vi "ConvertImage.vi"(11 "body":string) -> (3 "new picture":picture)   [LabVIEW 2019]
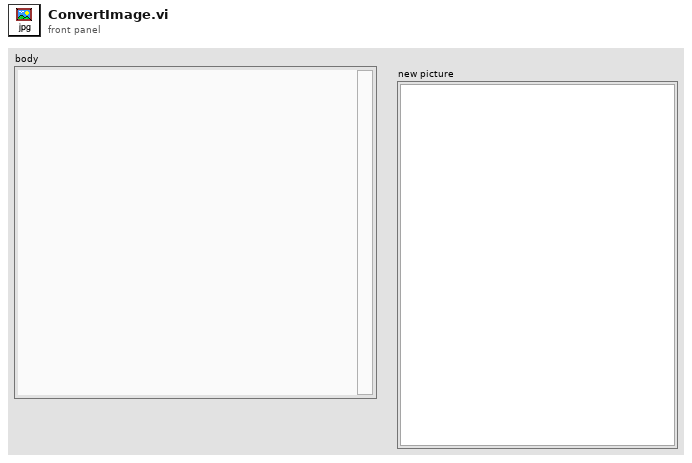
[diagram p1: front panel]
types:
  T1 = typedef "imagedata.ctl" = cluster{"image type":i32, "image depth":i32, "image":u8[], "mask":u8[], "colors":u32[], "Rectangle":cluster{"left":i16, "top":i16, "right":i16, "bottom":i16}}
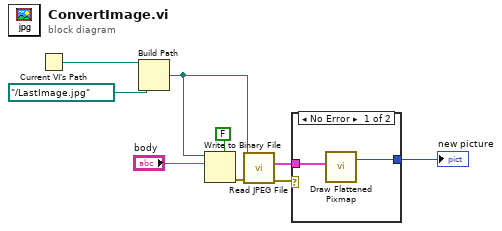
[diagram p0: block diagram]
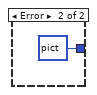
[diagram p2: hidden frame]
diagram:
  n1 = Current VI's Path() -> (path=w3:path)
  n2 = Build Path(base path=w3, name or relative path=path "../LastImage.jpg") -> (appended path=w2:path)
  n3 = Write to Binary File(file (use dialog)=w2, data="body", 5:FALSE ("prepend array or string size? (T)")) -> (error out=w9:errorcluster)  [unwired: 3 in, 2 out]
  n4 = call <vilib>:"Read JPEG File.vi"("error in (no error)"=w9, "path to JPEG file"=w2) -> ("error out"=w4:errorcluster, "image data"=w5:T1)  [unwired: 7 in, 1 out]
  n5 = case shown="No Error" w4 {
    tunnel: [w11 picture data[5B] ("new picture")] -> w7
    tunnel: w5 -> [w10 _]
    frame No Error {
      n6 = call <vilib>:"Draw Flattened Pixmap.vi"("image data"=w10) -> ("new picture"=w11:picture)  [unwired: 8 in]
    }
    frame Error {
    }
  }
  "new picture" <- w7
